vi "host.vi"() -> ()   [LabVIEW 2020]
uses:
  <vilib>/Analysis/Matrix/Datatypes/RealMatrix.ctl
  <vilib>/Analysis/baseanly.llb/Real A x B.vi
  <vilib>/Analysis/7linalg.llb/Real Cholesky Factorization.vi
  <vilib>/Analysis/7linalg.llb/Real Transpose Matrix.vi
  <vilib>/Analysis/baseanly.llb/Full Cholesky Factorization.vi
  <vilib>/Analysis/baseanly.llb/Full Real Matrix Cholesky Factorization.vi
  <vilib>/FPGAPlugInAG/cRIO-9035/niLvFpga_Open_cRIO-9035.vi
  <vilib>/rvi/interface/common/dynamic/niFpgaDynamicAddResources.vi
  <vilib>/Utility/error.llb/Error Cluster From Error Code.vi
  <vilib>/rvi/errors/niLvFpgaAdjustHostInterfaceError.vi
  <vilib>/FPGAPlugInAG/Dynamic/niLvFpga_Run_Dynamic.vi
  <vilib>/Analysis/Matrix/Numeric/Subtract/Subtract - RM,RM.vi
  <vilib>/FPGAPlugInAG/Dynamic/niLvFpga_Close_Dynamic.vi
  <vilib>/rvi/interface/nirviOpenFPGA/nirviOpenFPGA.xnode
  FPGA Bitfiles/labviewfpgacheck_FPGATarget_target_ofARWKwcoZM.lvbitx
  target.vi
  <vilib>/rvi/interface/nirviMethod/nirviMethod.xnode
  <vilib>/rvi/interface/nirviCloseFPGA/nirviCloseFPGA.xnode
  <vilib>/FPGAPlugInAG/Dynamic/niLvFpga_WriteFifo_Dynamic.vi
  <vilib>/rvi/errors/niLvFpgaMergeErrorWithErrorCode.vi
  <vilib>/FPGAPlugInAG/Dynamic/niLvFpga_ReadFifo_Dynamic.vi
  <vilib>/Analysis/NI_AALBase.lvlib
  <vilib>/Analysis/Matrix/NI_Matrix.lvlib
  <vilib>/Analysis/NI_AALPro.lvlib
panel:
  out "A x B":T1
  out "sum of error":dbl
  out "C - FPGA code":sgl[][](array[numeric])
  out "A":sgl[][](array[numeric])
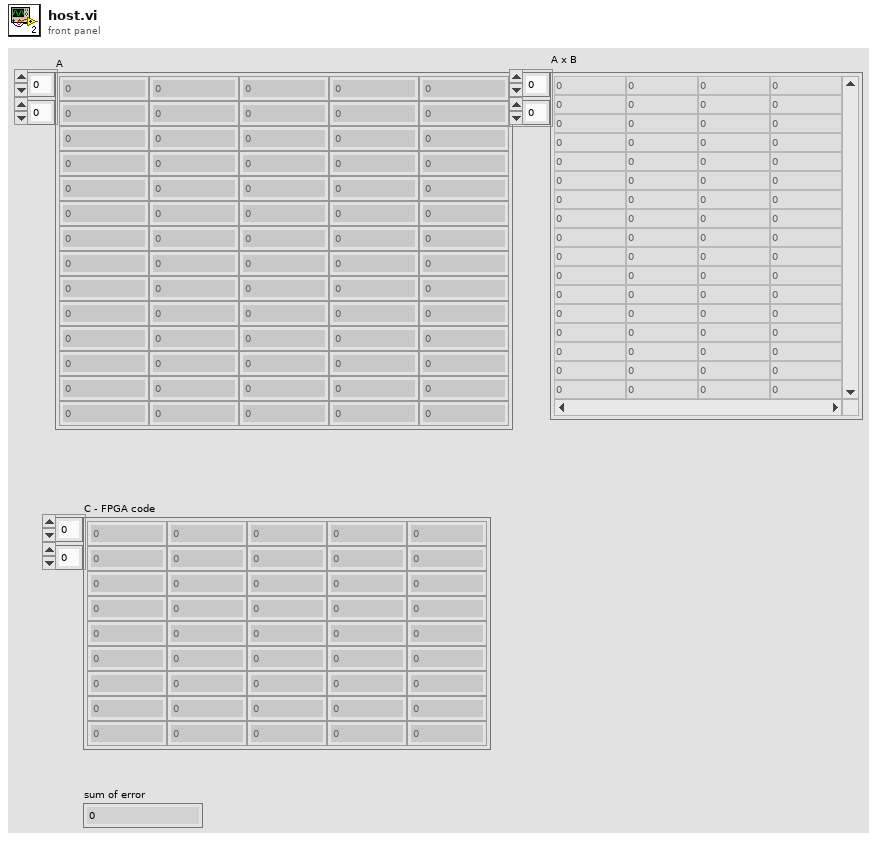
[diagram p1: front panel]
types:
  T1 = typedef "NI_Matrix.lvlib/RealMatrix.ctl" = dbl[][]
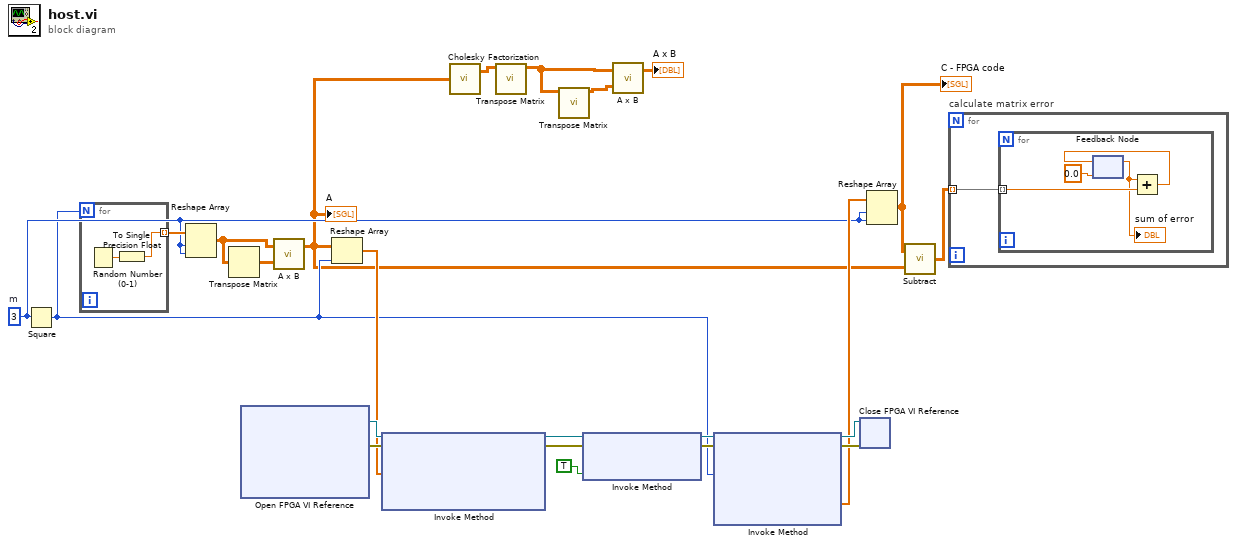
[diagram p0: block diagram]
diagram:
  w7 = 3  # m
  n1 = Square(x=w7) -> (x^2=w6:i32)
  n2 = for {
    N: w6 -> [_]
    tunnel: [w24] -> w10 mode=indexing
    n3 = Random Number (0-1)() -> (number: 0 to 1=w25:dbl)
    n4 = To Single Precision Float(number=w25) -> (single precision float=w24:sgl)
  }
  n5 = Reshape Array(w10, w7, w7) -> (w8:sgl[][])
  n6 = Transpose Matrix(1:w8) -> (0:w9:dbl[][])
  n7 = xnode "Open FPGA VI Reference"() -> ("FPGA VI Reference Out"=w22:refnum<k20>, "error out"=w21:errorcluster)  [unwired: 2 in]
  n8 = call-poly <vilib>:"A x B.vi"("B"=w9, "A"=w8) -> ("A x B"=w2:T1)  [unwired: 1 out]
  "A" <- w2
  n9 = Reshape Array(w2, w6) -> (w16:dbl[])
  n10 = xnode "Invoke Method"("FPGA VI Reference In"=w22, "error in"=w21, "Data"=w16) -> ("FPGA VI Reference Out"=w12:refnum<k20>, "error out"=w11:errorcluster)  [unwired: 1 in, 1 out]
  n11 = call-poly <vilib>:"Cholesky Factorization.vi"("A"=w2) -> ("Cholesky"=w5:T1)  [unwired: 1 out]
  n12 = call-poly <vilib>:"Transpose Matrix.vi"("Input Matrix"=w5) -> ("Matrix Transpose"=w1:T1)  [unwired: 9 in, 1 out]
  n13 = call-poly <vilib>:"Transpose Matrix.vi"("Input Matrix"=w1) -> ("Matrix Transpose"=w3:T1)  [unwired: 9 in, 1 out]
  n14 = xnode "Invoke Method"("FPGA VI Reference In"=w12, "error in"=w11, "Wait Until Done (F)"=TRUE) -> ("FPGA VI Reference Out"=w20:refnum<k20>, "error out"=w19:errorcluster)
  n15 = call-poly <vilib>:"A x B.vi"("B"=w3, "A"=w1) -> ("A x B"=→"A x B":T1)  [unwired: 1 out]
  n16 = xnode "Invoke Method"("FPGA VI Reference In"=w20, "error in"=w19, "Number of Elements"=w6) -> ("FPGA VI Reference Out"=w18:refnum<k20>, "error out"=w17:errorcluster, "Data"=w13:sgl[])  [unwired: 1 in, 1 out]
  n17 = xnode "Close FPGA VI Reference"("FPGA VI Reference In"=w18, "error in"=w17) -> ()  [unwired: 1 out]
  n18 = Reshape Array(w13, w7, w7) -> (w15:sgl[][])
  "C - FPGA code" <- w15
  n19 = call-poly <vilib>:"Subtract.vi"("Real Matrix B"=w2, "Real Matrix A"=w15) -> ("A - B"=w14:T1)
  n20 = for "calculate matrix error" {
    tunnel: w14 -> [w26] mode=indexing
    n21 = for {
      tunnel: w26 -> [w30] mode=indexing
      n22 = feedback #1(0.0) -> (w28:dbl)
      "sum of error" <- w28
      n23 = Add(x=w28, y=w30) -> (x+y=w29:dbl)
      n24 = feedback-in #1(w29) -> ()
    }
  }
